vi "Update Identity Plot (P-Ph-tau Graph).vi"(6 "Delta tau":bool, 8 "error in (no error)":errorcluster, 11 "XYGraph in":refnum<vi>) -> (0 "error out":errorcluster)   [LabVIEW 2019]
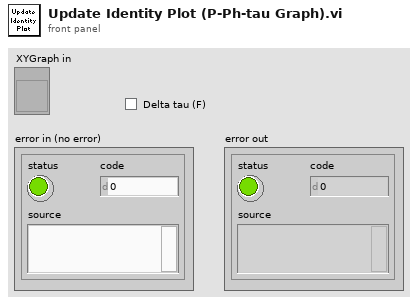
[diagram p1: front panel]
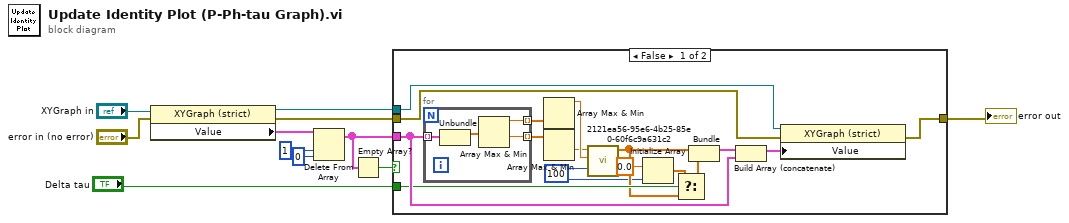
[diagram p0: block diagram]
diagram:
  n1 = property class="XYGraph (strict)"(reference="XYGraph in", error in="error in (no error)") -> (reference out=w3:refnum<vi>, error out=w4:errorcluster, "Value"=w7:cluster{"X Array":dbl[], "Y Array":dbl[]}[])
  n2 = Delete From Array(array=w7, length=1, index=0) -> (array with subset deleted=w10:cluster{"X Array":dbl[], "Y Array":dbl[]}[])  [unwired: 1 out]
  n3 = Empty Array?(array=w10) -> (empty?=w5:bool)
  n4 = case shown="False" w5 {
    tunnel: w10 -> [w23 _]
    tunnel: w4 -> [w20 w32]
    tunnel: w3 -> [w21 _]
    tunnel: [w18 w32] -> w2
    tunnel: "Delta tau" -> [w17 _]
    frame False {
      w15 = 100 ("# Steps (1)")
      n5 = for {
        tunnel: w23 -> [w31] mode=indexing
        tunnel: [w29] -> w26 mode=indexing
        tunnel: [w28] -> w27 mode=indexing
        n6 = Unbundle(w31) -> ("X Array"=w30:dbl[])  [unwired: 1 out]
        n7 = Array Max & Min(array=w30) -> (max value=w29:dbl, min value=w28:dbl)  [unwired: 2 out]
      }
      n8 = Array Max & Min(array=w26) -> (max value=w25:dbl)  [unwired: 3 out]
      n9 = Array Max & Min(array=w27) -> (min value=w24:dbl)  [unwired: 3 out]
      n10 = call "2121ea56-95e6-4b25-85e0-60f6c9a631c2.vi"("# Steps (1)"=w15, "End (1)"=w25, "Start (0)"=w24) -> ("Ramp"=w16:dbl[])  [unwired: 6 in, 2 out]
      n11 = Initialize Array(0.0 ("element"), w15) -> (w14:dbl[])
      n12 = Select(t=w14, s=w17, f=w16) -> (s? t:f=w13:dbl[])
      n13 = Bundle("Ramp"=w16, "Ramp"=w13) -> (w22:cluster{"Ramp":dbl[], "Ramp":dbl[]})  [unwired: 1 in]
      n14 = Build Array (concatenate)(w22, w23) -> (w19:cluster{"X Array":dbl[], "Y Array":dbl[]}[])
      n15 = property class="XYGraph (strict)"(reference=w21, error in=w20, "Value"=w19) -> (error out=w18:errorcluster)  [unwired: 1 out]
    }
    frame True {
    }
  }
  "error out" <- w2
